vi "createTopicClusterControlRefCtrl.vi"(8 "error in (no error)":errorcluster, 11 "PolymorphicInstance in":refnum<class "PolymorphicInstance.lvclass">) -> (0 "error out":errorcluster, 3 "PolymorphicInstance out":refnum<class "PolymorphicInstance.lvclass">)   [LabVIEW 2013, in "PolymorphicInstance.lvclass"]
uses:
  PolymorphicInstance.lvclass
  <vilib>/Utility/miscctls.llb/LVPositionTypeDef.ctl
  PolymorphicInstance.lvclass/PolymorphicInstance.ctl
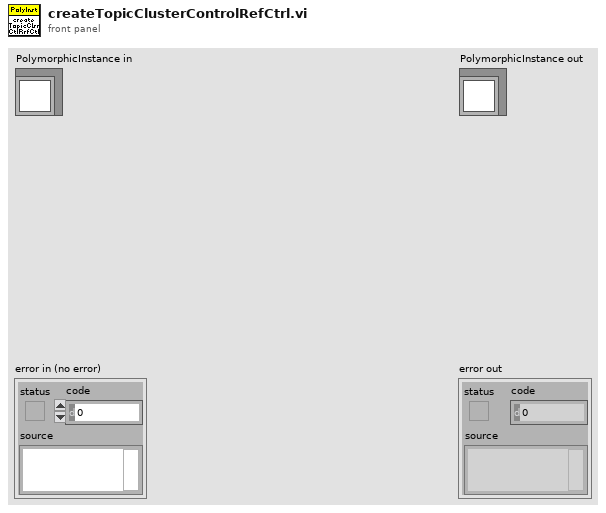
[diagram p1: front panel]
types:
  T1 = typedef "LVPositionTypeDef.ctl" = cluster{"Left":i32, "Top":i32}
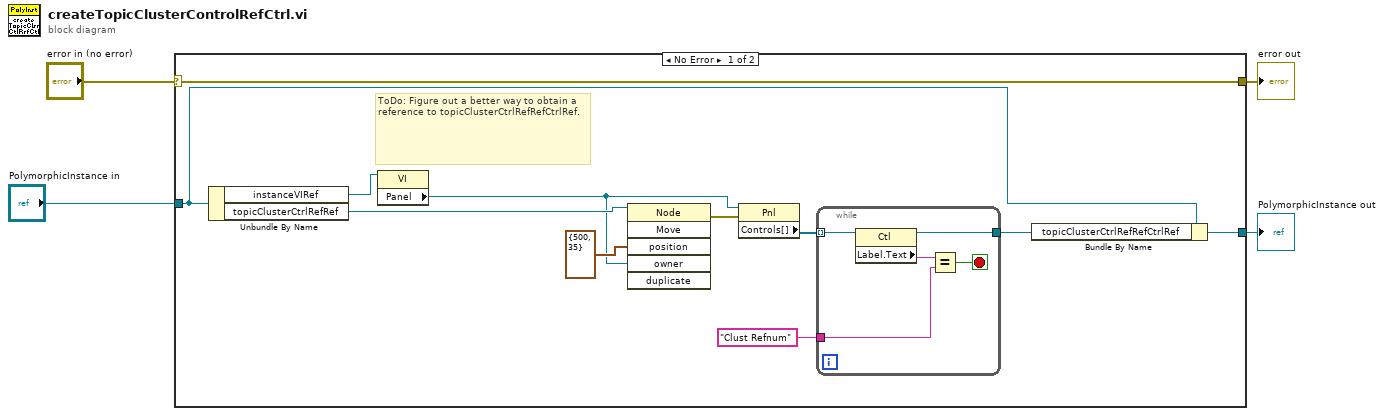
[diagram p0: block diagram]
diagram:
  n1 = case shown="No Error" "error in (no error)" {
    selector: "error in (no error)" -> [w15 w22]
    tunnel: [w15 w22] -> w3
    tunnel: [w5 w21] -> w1
    tunnel: "PolymorphicInstance in" -> [w6 w21]
    frame No Error {
      # "ToDo: Figure out a better way to obtain a reference to topicClusterCtrlRefRefCtrlRef."
      n2 = Unbundle By Name(w6) -> ("instanceVIRef"=w11:refnum<vi>, "topicClusterCtrlRefRef"=w10:refnum<vi>)
      n3 = property class="VI"(reference=w11) -> ("Panel"=w8:refnum<vi>)  [unwired: 1 in, 2 out]
      n4 = invoke class="Node" method="Move"(reference=w10, "position"=T1 {"Left"=500, "Top"=35}, "owner"=w8) -> (error out=w9:errorcluster)  [unwired: 3 in, 5 out]
      n5 = property class="Pnl"(reference=w8, error in=w9) -> ("Controls[]"=w14:refnum<vi>[])  [unwired: 2 out]
      n6 = while {
        tunnel: w14 -> [w20] mode=indexing
        tunnel: "Clust Refnum" ("Label.Text") -> [w18]
        tunnel: [w16] -> w7
        stop <- w17 stop-if-true
        n7 = property class="Ctl"(reference=w20) -> (reference out=w16:refnum<vi>, "Label.Text"=w19:string)  [unwired: 1 in, 1 out]
        n8 = Equal?(x=w19, y=w18) -> (x = y?=w17:bool)
      }
      n9 = Bundle By Name(cluster=w6, "topicClusterCtrlRefRefCtrlRef"=w7) -> (w5:refnum<class "PolymorphicInstance.lvclass">)
    }
    frame Error {
    }
  }
  "error out" <- w3
  "PolymorphicInstance out" <- w1
